vi "auto measurement.vi"(7 "ref. line [dB]":dbl, 8 "error in":errorcluster, 10 "App Data":T1, 11 "XYGraph in":refnum<vi>) -> (0 "error out":errorcluster)   [LabVIEW 2014]
uses:
  Controls/App Data.ctl
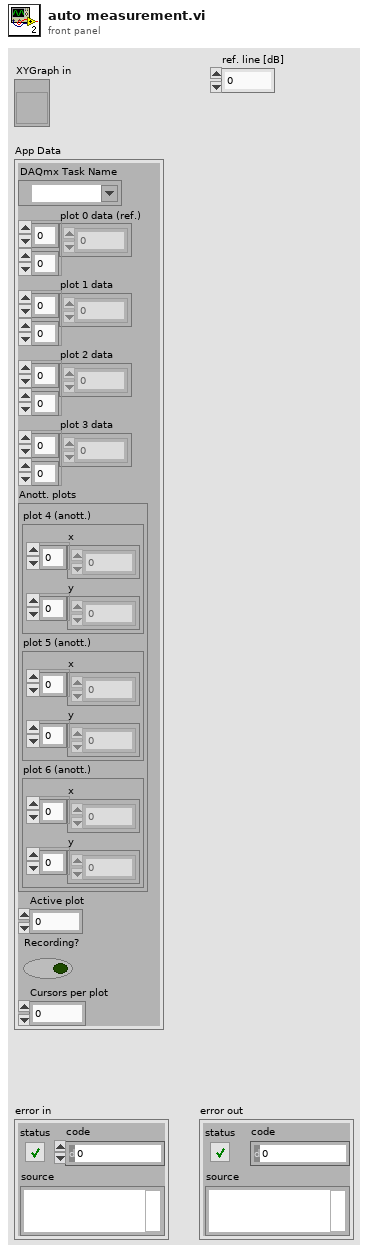
[diagram p1: front panel]
types:
  T1 = typedef "App Data.ctl" = cluster{"DAQmx Task Name":refnum<k21>, "plot 0 data (ref.)":dbl[][], "plot 1 data":dbl[][], "plot 2 data":dbl[][], "plot 3 data":dbl[][], "Anott. plots":cluster{"plot 4 (anott.)":cluster{"x":dbl[], "y":dbl[]}, "plot 5 (anott.)":cluster{"x":dbl[], "y":dbl[]}, "plot 6 (anott.)":cluster{"x":dbl[], "y":dbl[]}}, "Active plot":u32, "Recording?":bool, "Cursors per plot":i32}
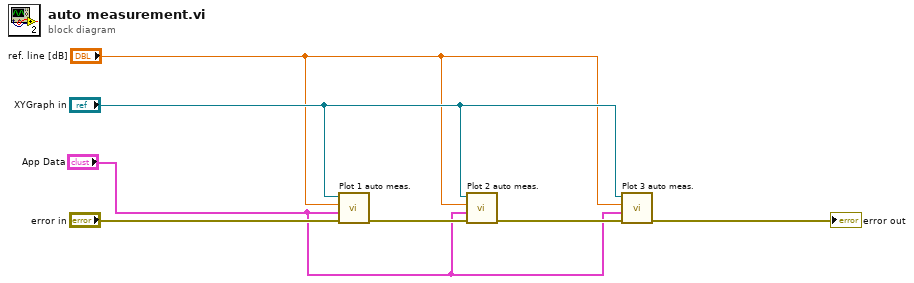
[diagram p0: block diagram]
diagram:
  n1 = call "Plot 1 auto meas..vi"("error in (no error)"="error in", "App Data"="App Data", "ref. line [dB]"="ref. line [dB]", "XYGraph in"="XYGraph in") -> ("error out"=w6:errorcluster)  [unwired: 7 in]
  n2 = call "Plot 2 auto meas..vi"("error in (no error)"=w6, "App Data"="App Data", "ref. line [dB]"="ref. line [dB]", "XYGraph in"="XYGraph in") -> ("error out"=w5:errorcluster)  [unwired: 7 in]
  n3 = call "Plot 3 auto meas..vi"("error in (no error)"=w5, "App Data"="App Data", "ref. line [dB]"="ref. line [dB]", "XYGraph in"="XYGraph in") -> ("error out"=→"error out":errorcluster)  [unwired: 7 in]
